vi "Release Registry Ownership.vi"(11 "Token":string) -> ()   [LabVIEW 2014, in "UniqueName.lvlib" / "UniqueName.lvclass"]
uses:
  UniqueName.lvclass
  Command.ctl
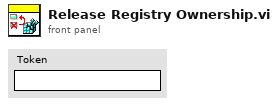
[diagram p1: front panel]
types:
  T1 = typedef "UniqueName.lvlib/UniqueName.lvclass/Command.ctl" = enum16{"Get", "Get All", "Set", "Delete", "Get Status", "Init", "Reserve Ownership", "Release Ownership", "Lock", "Unlock"}
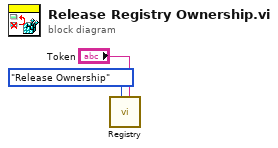
[diagram p0: block diagram]
diagram:
  n1 = call "Registry.vi"("Token"="Token", "Command (Get)"=Command."Release Ownership") -> ()  [unwired: 5 in, 5 out]
